vi "Reliability Indicator.vi"(8 "error in (no error)":errorcluster, 9 "Reliability Code":i32, 11 "VISA resource name":refnum<visa-resource-name>) -> (0 "error out":errorcluster, 1 "Reliability Message":string, 3 "VISA resource name out":refnum<visa-resource-name>)   [LabVIEW 2015, in "Rohde&Schwarz CMXP GPRF.lvlib"]
doc: "This VI converts Reliability Code you enter into a human-readable message."
uses:
  <instrlib>/Rohde&Schwarz CMXP GPRF/Rohde&Schwarz CMXP GPRF.lvlib
  <instrlib>/Rohde&Schwarz CMXP GPRF/Private/rsidr_core.llb/type_Error_Codes.ctl
  <instrlib>/Rohde&Schwarz CMXP GPRF/Private/rsidr_core.llb/rsidr_core.lvlib
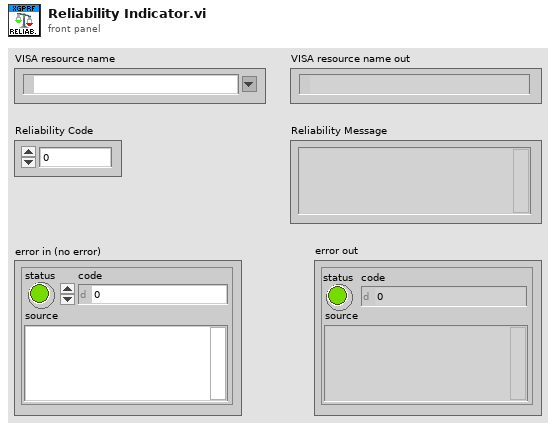
[diagram p1: front panel]
types:
  T1 = typedef "Rohde&Schwarz CMXP GPRF.lvlib/rsidr_core.lvlib/type_Error_Codes.ctl" = enum16{"No_error", "VISA_err_ResourceNotFound", "VISA_err_Timeout", "VISA_warn_MoreDataAvailable", "RS_err_MissingCallback", "RS_err_InvalidAttribute", "RS_err_InvalidValue", "RS_err_UnknownResource", "RS_err_AlreadyInitialized", "RS_err_InstrumentStatus", "RS_err_BadRepCapName", "RS_err_TypesMismatch", "RS_err_ValueNotSupported", "RS_err_InvalidRngTable", "RS_err_IDqueryFail", "RS_err_UnexpResponse", "VISA_warn_ConfigNotLoaded", "RS_err_AttributeNotReadable", "RS_err_AttributeNotWritable", "RS_err_InstrumentType", "RS_err_InstrumentOption", "VISA_err_InvalidSize", "RS_err_ReliabilityIndicator", "VISA_warn_UnknownStatus", "VISA_warn_TermCharRead", "VISA_err_IO_error", "RS_err_FunctionNotSupported", "VISA_warn_QueueEmpty"}
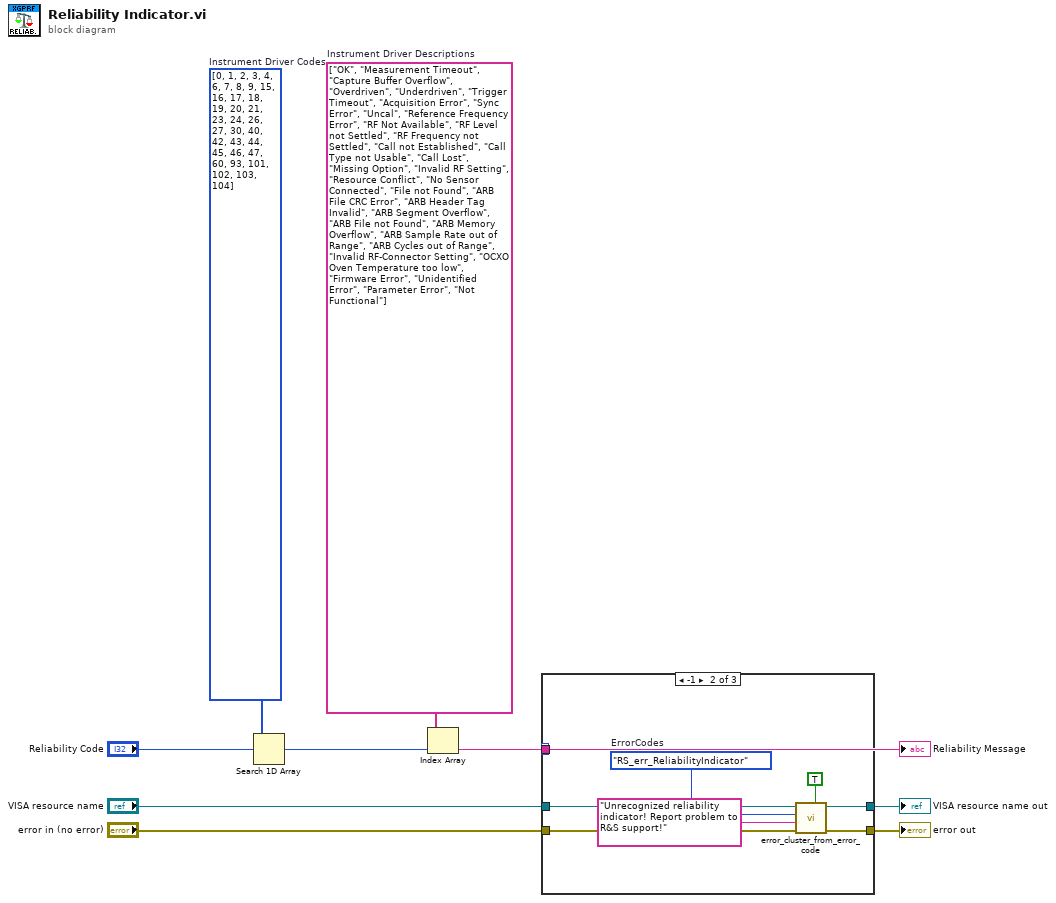
[diagram p0: block diagram]
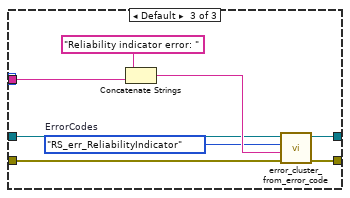
[diagram p3: hidden frame]
diagram:
  w1 = i32[] [0, 1, 2, 3, 4, 6, 7, 8, 9, 15, 16, 17, 18, 19, 20, 21, 23, 24, 26, 27, 30, 40, 42, 43, 44, 45, 46, 47, 60, 93, 101, 102, 103, 104]  # Instrument Driver Codes
  w2 = string[] ["OK", "Measurement Timeout", "Capture Buffer Overflow", "Overdriven", "Underdriven", "Trigger Timeout", "Acquisition Error", "Sync Error", "Uncal", "Reference Frequency Error", "RF Not Available", "RF Level not Settled", "RF Frequency not Settled", "Call not Established", "Call Type not Usable", "Call Lost", "Missing Option", "Invalid RF Setting", "Resource Conflict", "No Sensor Connected", "File not Found", "ARB File CRC Error", "ARB Header Tag Invalid", "ARB Segment Overflow", "ARB File not Found", "ARB Memory Overflow", "ARB Sample Rate out of Range", "ARB Cycles out of Range", "Invalid RF-Connector Setting", "OCXO Oven Temperature too low", "Firmware Error", "Unidentified Error", "Parameter Error", "Not Functional"]  # Instrument Driver Descriptions
  n1 = Search 1D Array(1D array=w1, element="Reliability Code") -> (index of element=w3:i32)  [unwired: 1 in]
  n2 = Index Array(array=w2, index=w3) -> (element=w8:string)
  "Reliability Message" <- w8
  n3 = case shown="-1" w3 {
    tunnel: "error in (no error)" -> [w11 w16 w23]
    tunnel: [w11 w14 w21] -> w5
    tunnel: w8 -> [_ _ w24]
    tunnel: "VISA resource name" -> [w10 w15 w22]
    tunnel: [w10 w13 w20] -> w4
    frame 0 {
    }
    frame -1 {
      w12 = type_Error_Codes."RS_err_ReliabilityIndicator"  # ErrorCodes
      n4 = call <instrlib>:"error_cluster_from_error_code.vi"("Is Warning (False)"=TRUE ("is warning? (False)"), "error in"=w16, "Error Message (\"\")"="Unrecognized reliability indicator! Report problem to R&S support!" ("error message (\"\")"), "Error Enum in"=w12, "VISA resource name"=w15) -> ("error out"=w14:errorcluster, "VISA resource name out"=w13:refnum<visa-resource-name>)  [unwired: 5 in]
    }
    frame Default {
      w19 = type_Error_Codes."RS_err_ReliabilityIndicator"  # ErrorCodes
      n5 = Concatenate Strings("Reliability indicator error: " ("error message (\"\")"), w24) -> (w25:string)
      n6 = call <instrlib>:"error_cluster_from_error_code.vi"("error in"=w23, "Error Message (\"\")"=w25, "Error Enum in"=w19, "VISA resource name"=w22) -> ("error out"=w21:errorcluster, "VISA resource name out"=w20:refnum<visa-resource-name>)  [unwired: 6 in]
    }
  }
  "VISA resource name out" <- w4
  "error out" <- w5
